vi "PB_Set.vi"(0 "Set Master":bool=TRUE, 1 "Master Output Bits":bool[](array[boolean])=[FALSE, FALSE, FALSE, FALSE, FALSE, FALSE, FALSE, FALSE, FALSE, FALSE, FALSE, FALSE, FALSE, FALSE, FALSE, TRUE, TRUE, TRUE, FALSE, FALSE, FALSE, FALSE, FALSE, FALSE], 2 "Set Slave":bool, 3 "Slave Output Bits":bool[](array[boolean])=[FALSE, FALSE, FALSE, FALSE, FALSE, FALSE, FALSE, FALSE, FALSE, FALSE, FALSE, FALSE, FALSE, FALSE, FALSE, FALSE, FALSE, FALSE, FALSE, FALSE, FALSE, FALSE, FALSE, FALSE], 4 "error in":errorcluster) -> (5 "Master Data Bits":u32=229727 format="%.0x", 6 "Slave Data Bits":u32=229727 format="%.0x", 7 "error out":errorcluster)   [LabVIEW 2013]
uses:
  DeviceVIs/Pulseblaster/PulseBlaster.lvlib
panel:
  # "Master PB"
  # "Slave PB"
  # "0"
  # "8"
  # "12"
  # "4"
  # "16"
  # "20"
  # "0"
  # "8"
  # "12"
  # "4"
  # "16"
  # "20"
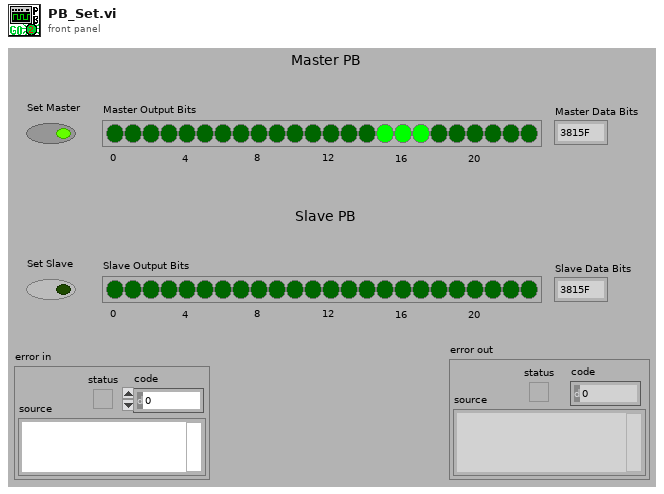
[diagram p1: front panel]
types:
  T1 = cluster{"Output Bits":u32, "Data Field":u32, "OP Code":u8, "Delay Count":u32}[]
  T2 = cluster{"Output Bits":u32, "Data Field":u32, "OP Code":u8, "Delay Count":u64}[]
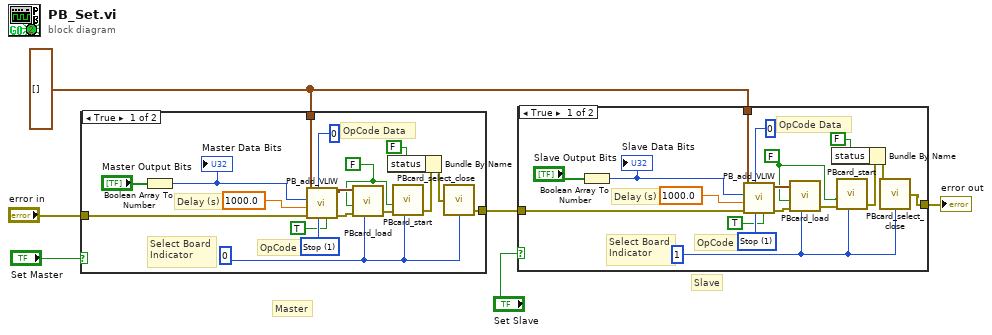
[diagram p0: block diagram]
diagram:
  w1 = T1 [] ("VLIW Array In")
  # "Slave"
  # "Master"
  n1 = case shown="True" "Set Master" {
    tunnel: [w12 w24] -> w3
    tunnel: "error in" -> [w18 w24]
    tunnel: w1 -> [w17 _]
    frame True {
      w8 = 0
      w13 = FALSE
      w21 = u8 1 items=["Continue", "Stop", "Loop", "End Loop", "Jump", "Return", "Go To", "Long Delay"] ("OP code")
      # "OpCode"
      # "OpCode Data"
      # "Delay (s)"
      # "Select Board\nIndicator"
      n2 = Boolean Array To Number(Boolean array="Master Output Bits") -> (number=w19:u32)
      "Master Data Bits" <- w19
      n3 = call "PB_add_VLIW.vi"("Use Global (F)?"=TRUE, "OP code"=w21, "Data Field"=u32 0, "error in (no error)"=w18, "Delay"=1000.0, "Digital Bits"=w19, "VLIW Array In"=w17) -> ("error out"=w16:errorcluster, "VLIW Array Out"=w15:T2)  [unwired: 2 in, 1 out]
      n4 = call "PBcard_load.vi"("PulseBlaster\nVLIW Array"=w15, "Memory"=w13, "error in"=w16, "Select Board Indicator"=w8) -> ("error out"=w14:errorcluster)  [unwired: 1 in, 2 out]
      n5 = call "PBcard_start.vi"("Memory"=w13, "error in (no error)"=w14, "Select Board\nIndicator"=w8) -> ("error out"=w11:errorcluster)  [unwired: 1 in, 3 out]
      n6 = Bundle By Name(cluster=w11, "status"=FALSE) -> (w10:errorcluster)
      n7 = call "PBcard_select_close.vi"("error in (no error)"=w10, "Select Board Indicator"=w8) -> ("error out"=w12:errorcluster)
    }
    frame False {
    }
  }
  n8 = case shown="True" "Set Slave" {
    tunnel: [w30 w42] -> w4
    tunnel: w3 -> [w38 w42]
    tunnel: w1 -> [w37 _]
    frame True {
      w26 = 1
      w39 = u8 1 items=["Continue", "Stop", "Loop", "End Loop", "Jump", "Return", "Go To", "Long Delay"] ("OP code")
      w31 = FALSE
      # "OpCode"
      # "OpCode Data"
      # "Delay (s)"
      # "Select Board\nIndicator"
      n9 = Boolean Array To Number(Boolean array="Slave Output Bits") -> (number=w36:u32)
      "Slave Data Bits" <- w36
      n10 = call "PB_add_VLIW.vi"("Use Global (F)?"=TRUE, "OP code"=w39, "Data Field"=u32 0, "error in (no error)"=w38, "Delay"=1000.0, "Digital Bits"=w36, "VLIW Array In"=w37) -> ("error out"=w34:errorcluster, "VLIW Array Out"=w33:T2)  [unwired: 2 in, 1 out]
      n11 = call "PBcard_load.vi"("PulseBlaster\nVLIW Array"=w33, "Memory"=w31, "error in"=w34, "Select Board Indicator"=w26) -> ("error out"=w32:errorcluster)  [unwired: 1 in, 2 out]
      n12 = call "PBcard_start.vi"("Memory"=w31, "error in (no error)"=w32, "Select Board\nIndicator"=w26) -> ("error out"=w28:errorcluster)  [unwired: 1 in, 3 out]
      n13 = Bundle By Name(cluster=w28, "status"=FALSE) -> (w27:errorcluster)
      n14 = call "PBcard_select_close.vi"("error in (no error)"=w27, "Select Board Indicator"=w26) -> ("error out"=w30:errorcluster)
    }
    frame False {
    }
  }
  "error out" <- w4
